vi "Hi_Tec_Control.vi"(0 "Carrier 1 Voltage":dbl(knob) min=0.0 max=5.0 scale=0.0..5.0 scale format="%.1f", 1 "Carrier 2 Voltage":dbl(knob) min=0.0 max=5.0 scale=0.0..5.0 scale format="%.1f", 2 "Trace Voltage":dbl(knob) min=0.0 max=5.0 scale=0.0..5.0 scale format="%.1f", 4 "Client Name":string) -> (5 "Scan Comments":string)   [LabVIEW 2014]
uses:
  Anemometry/Anemometry Sub Vis/Controls/In_Range.ctl
  ADAM Client/Sub VIs/ADAM Controls/Update_scan_value.ctl
panel:
  out "Second stage":dbl[][](graph)
  out "First stage":dbl[][](graph)
  out "Increasing trace":bool
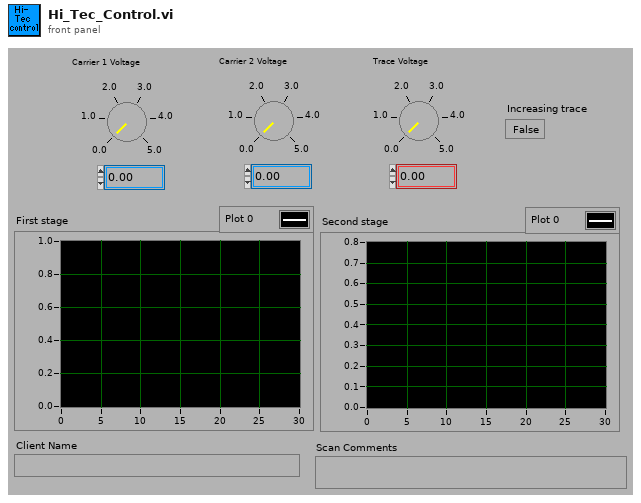
[diagram p1: front panel]
types:
  T1 = typedef "In_Range.ctl" = enum16{"%", "±", "% & ±"}
  T2 = typedef "Update_scan_value.ctl" = cluster{"Channel Name":string, "New Value":dbl}
  T3 = enum16{"Append to Global", "Read Global then Clear"}
  T4 = typedef "Ch_description_ADAM.ctl" = cluster{"Ch Name":string, "Type":T5, "Function":T6, "Ch State":T7, "Calibration type":T8, "A":dbl, "B":dbl, "C":dbl, "D":dbl, "Comments":string, "Address":T9, "String":string, "Duty":u16}
  T5 = typedef "Module_type_ADAM.ctl" = string
  T6 = typedef "Function_ADAM.ctl" = enum16{"Analogue Input", "Digital Input", "Event counter", "Event rate", "Analogue Output", "Digital Output", "Relay Output"}
  T7 = typedef "Channel_State.ctl" = enum16{"On", "Off", "Always On", "Always Off"}
  T8 = typedef "Calib_type_ADAM.ctl" = enum16{"Raw", "Bx + A", "Cx^2 + Bx + A", "Dx^3 + Cx^2 + Bx + A", "In Band", "Hi-Tec Q", "Hi-Tec M_dot", "Text"}
  T9 = typedef "Address.ctl" = cluster{"Main":i32, "Ch.":i32, "Sub":i32, "Port Name":string}
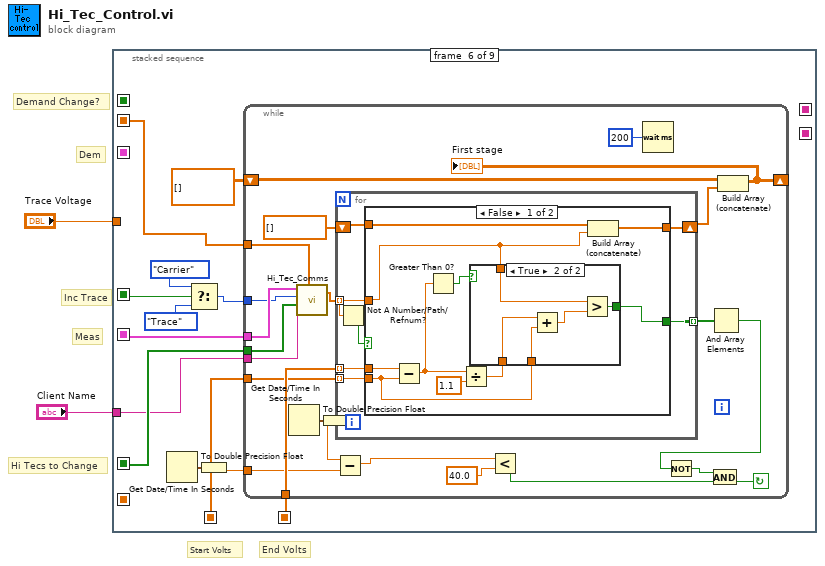
[diagram p0: block diagram]
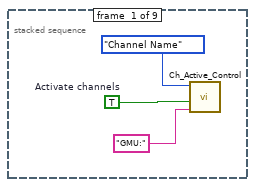
[diagram p2: hidden frame]
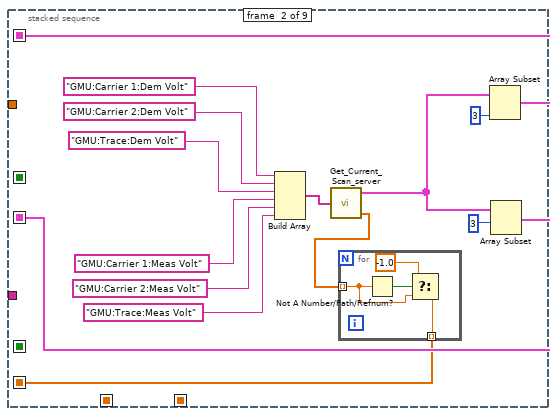
[diagram p3: hidden frame]
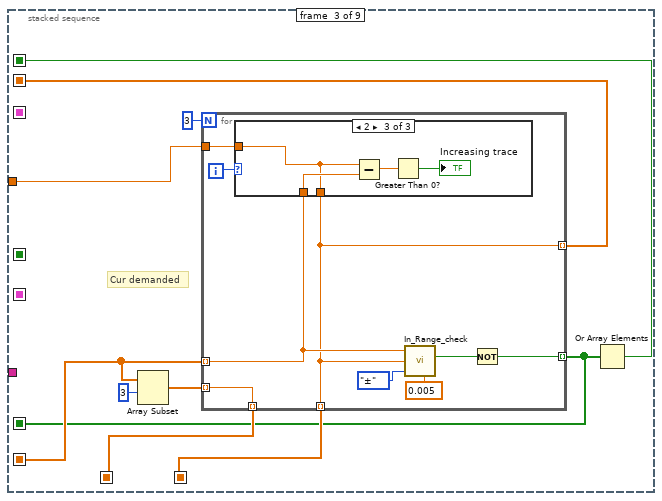
[diagram p4: hidden frame]
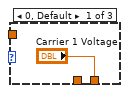
[diagram p5: hidden frame]
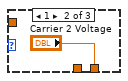
[diagram p6: hidden frame]
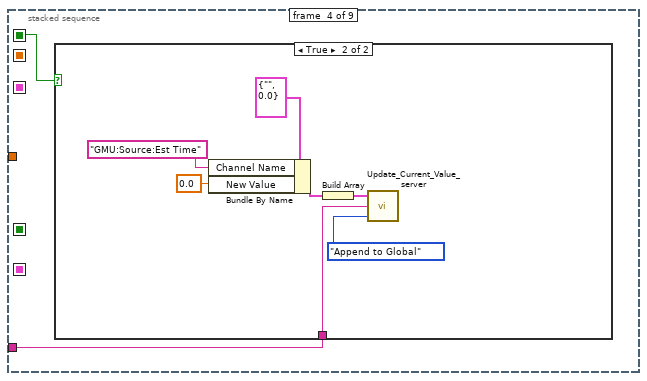
[diagram p7: hidden frame]
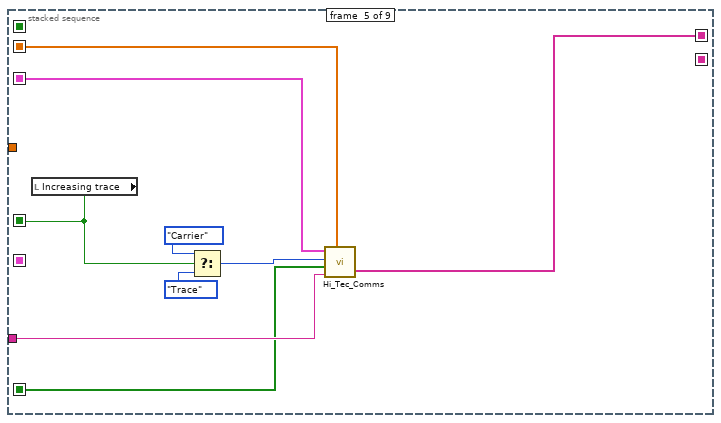
[diagram p9: hidden frame]
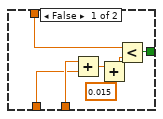
[diagram p10: hidden frame]
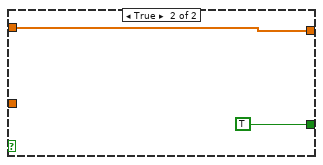
[diagram p11: hidden frame]
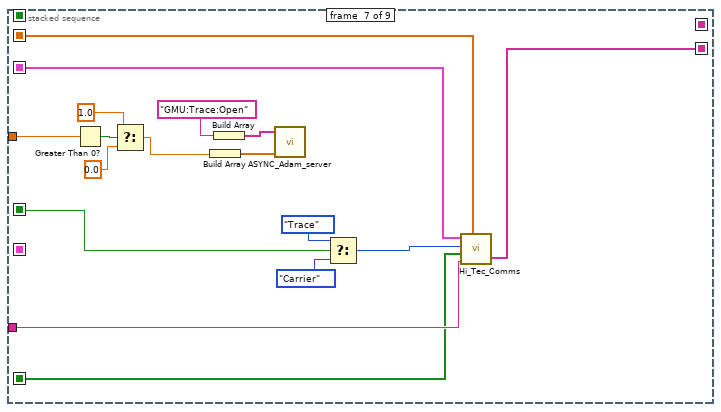
[diagram p12: hidden frame]
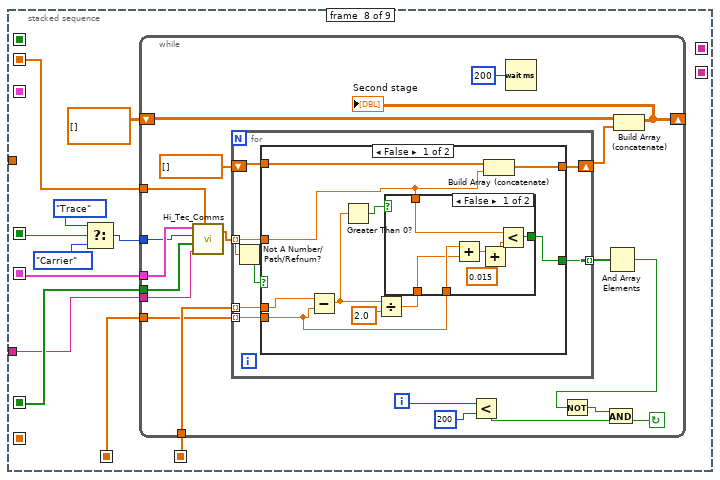
[diagram p13: hidden frame]
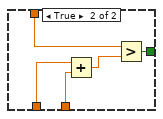
[diagram p14: hidden frame]
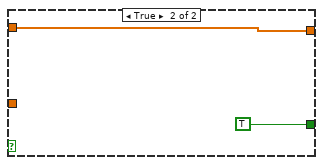
[diagram p15: hidden frame]
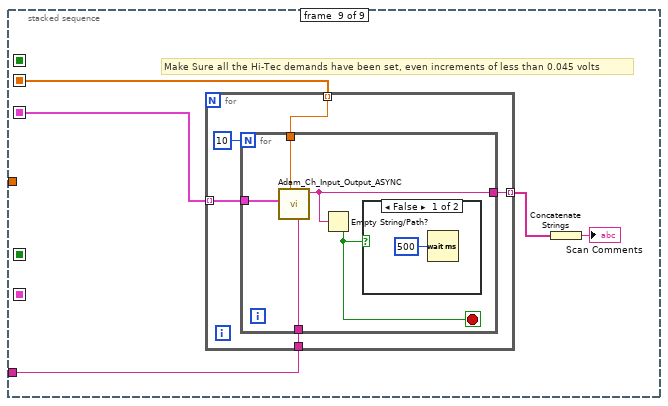
[diagram p16: hidden frame]
diagram:
  # "Dem"
  # "Demand Change?"
  # "End Volts"
  # "Start Volts"
  # "Inc Trace"
  # "Meas"
  # "Hi Tecs to Change"
  n1 = stacked-sequence {
    seq-local: [_ w14 _ _ _ _ _ _ _] -> [_ _ _ _ w60 _ w136 _ w216]
    seq-local: [_ w6 _ _ _ _ _ _ _] -> [_ _ w30 _ _ _ _ _ _]
    seq-local: [_ _ w27 _ _ _ _ _ _] -> [_ _ _ _ w59 w79 w135 w161 _]
    seq-local: [_ w13 _ _ _ _ _ _ _] -> [_ _ _ _ _ w75 _ w157 _]
    seq-local: [_ _ _ _ w66 _ _ _ _] -> [_ _ _ _ _ w76 w150 w158 _]
    seq-local: [_ _ w33 _ _ _ _ _ _] -> [_ _ _ _ _ w72 _ w154 _]
    seq-local: [_ _ w32 _ _ _ _ _ _] -> [_ _ _ _ _ w73 _ w155 _]
    seq-local: [_ _ w26 _ _ _ _ _ _] -> [_ _ _ w49 _ _ _ _ _]
    seq-local: [_ _ w24 _ _ _ _ _ _] -> [_ _ _ _ w61 w67 w137 w151 w215]
    seq-local: [_ _ _ _ w58 _ _ _ _] -> [_ _ _ _ _ _ _ _ _]
    seq-local: [_ _ _ _ _ _ w134 _ _] -> [_ _ _ _ _ _ _ _ _]
    tunnel: "Client Name" -> [_ _ _ w50 w62 w69 w146 w152 w217]
    tunnel: "Trace Voltage" -> [_ _ w25 _ _ _ w145 _ _]
    frame #0 {
      w3 = TRUE  # Activate channels
      n2 = call "Ch_Active_Control.vi"("Match"="GMU:", "Activate Channels?"=w3, "Control on"=enum16{"Channel Name", "Main Address"}."Channel Name") -> ()  [unwired: 1 in, 2 out]
    }
    frame #1 {
      n3 = Build Array("GMU:Carrier 1:Dem Volt", "GMU:Carrier 2:Dem Volt", "GMU:Trace:Dem Volt", "GMU:Carrier 1:Meas Volt", "GMU:Carrier 2:Meas Volt", "GMU:Trace:Meas Volt") -> (w19:string[])
      n4 = call "Get_Current_Scan_server.vi"("Desired Channels"=w19) -> ("Ch Description Array"=w12:T4[], "Numerical Values"=w7:dbl[])  [unwired: 1 out]
      n5 = for {
        tunnel: w7 -> [w22] mode=indexing
        tunnel: [w21] -> w6 mode=indexing
        n6 = Not A Number/Path/Refnum?(number/path/refnum=w22) -> (NaN/Path/Refnum?=w23:bool)
        n7 = Select(t=-1.0, s=w23, f=w22) -> (s? t:f=w21:dbl)
      }
      n8 = Array Subset(array=w12, length=3 ("Array Length")) -> (w14:T4[])  [unwired: 1 in]
      n9 = Array Subset(array=w12, index=3 ("Array Length")) -> (w13:T4[])  [unwired: 1 in]
    }
    frame #2 {
      # "Cur demanded"
      n10 = Array Subset(array=w30, index=3 ("Array Index")) -> (w28:dbl[])  [unwired: 1 in]
      n11 = for {
        N: 3 -> [_]
        tunnel: w30 -> [w37] mode=indexing
        tunnel: [w40] -> w33 mode=indexing
        tunnel: [w34] -> w32 mode=indexing
        tunnel: [w41] -> w27 mode=indexing
        tunnel: w28 -> [w40] mode=indexing
        tunnel: w25 -> [w35]
        tunnel: [w34] -> w24 mode=indexing
        i -> [w42]
        n12 = case shown="2" w42 {
          tunnel: ["Carrier 1 Voltage" "Carrier 2 Voltage" w45] -> w34
          tunnel: w37 -> [_ _ w48]
          tunnel: w35 -> [_ _ w45]
          frame 0, Default {
          }
          frame 1 {
          }
          frame 2 {
            n13 = Subtract(x=w45, y=w48) -> (x-y=w47:dbl)
            n14 = Greater Than 0?(x=w47) -> (x > 0?=→"Increasing trace":bool)
          }
        }
        n15 = call "In_Range_check.vi"("±"=0.005 ("%"), "Mode"=In_Range."±", "Value"=w34, "Setpoint"=w37) -> ("In Range"=w36:bool)  [unwired: 1 in, 2 out]
        n16 = Not(x=w36) -> (.not. x?=w41:bool)
      }
      n17 = Or Array Elements(Boolean array=w27) -> (logical OR=w26:bool)
    }
    frame #3 {
      n18 = case shown="True" w49 {
        tunnel: w50 -> [_ w57]
        frame False {
        }
        frame True {
          n19 = Bundle By Name(cluster=T2 {"Channel Name"="", "New Value"=0.0} ("Update Scan Value Cluster"), "Channel Name"="GMU:Source:Est Time", "New Value"=0.0 ("Bundle Element")) -> (w52:T2)
          n20 = Build Array(w52) -> (w51:T2[])
          n21 = call "Update_Current_Value_server.vi"("Mode"=T3."Append to Global", "Client HD name"=w57, "Update array in"=w51) -> ()  [unwired: 1 out]
        }
      }
    }
    frame #4 {
      n22 = local read "Increasing trace"() -> (w66:bool)
      n23 = Select(t=enum16{"Carrier", "Trace"}."Carrier" ("Type"), s=w66, f=enum16{"Carrier", "Trace"}."Trace" ("Type")) -> (s? t:f=w63:enum16{"Carrier", "Trace"})
      n24 = call "Hi_Tec_Comms.vi"("Ch Description Array"=w60, "Type"=w63, "Hi Tec's To Change"=w59, "Client Name"=w62, "Dem Volts"=w61) -> ("Scan comments"=w58:string[])  [unwired: 1 out]
    }
    frame #5 {
      n25 = Get Date/Time In Seconds() -> (seconds since 1Jan1904=w68:timestamp)
      n26 = Select(t=enum16{"Carrier", "Trace"}."Carrier" ("Type"), s=w76, f=enum16{"Carrier", "Trace"}."Trace" ("Type")) -> (s? t:f=w74:enum16{"Carrier", "Trace"})
      n27 = To Double Precision Float(number=w68) -> (double precision float=w70:dbl)
      n28 = while {
        tunnel: w69 -> [w83]
        tunnel: w70 -> [w86]
        shift-left: dbl[][] [] -> [w92]
        shift-right: [w91] -> _
        tunnel: w72 -> [w99]
        tunnel: w73 -> [w100]
        tunnel: w74 -> [w101]
        tunnel: w75 -> [w102]
        tunnel: w79 -> [w93]
        tunnel: w67 -> [w80]
        stop <- w88 continue-if-true
        n29 = Get Date/Time In Seconds() -> (seconds since 1Jan1904=w82:timestamp)
        n30 = call "Hi_Tec_Comms.vi"("Ch Description Array"=w102, "Type"=w101, "Hi Tec's To Change"=w93, "Client Name"=w83, "Dem Volts"=w80) -> ("Outputs"=w98:dbl[])  [unwired: 1 out]
        n31 = To Double Precision Float(number=w82) -> (double precision float=w87:dbl)
        n32 = Subtract(x=w87, y=w86) -> (x-y=w85:dbl)
        n33 = for {
          tunnel: w100 -> [w109] mode=indexing
          tunnel: w99 -> [w108] mode=indexing
          tunnel: w98 -> [w104] mode=indexing
          tunnel: [w107] -> w97 mode=indexing
          shift-right: [w105] -> w94
          shift-left: dbl[] [] -> [w106]
          n34 = Not A Number/Path/Refnum?(number/path/refnum=w104) -> (NaN/Path/Refnum?=w103:bool)
          n35 = case shown="False" w103 {
            tunnel: w109 -> [w116 _]
            tunnel: w108 -> [w112 _]
            tunnel: w104 -> [w111 _]
            tunnel: [w110 TRUE] -> w107
            tunnel: w106 -> [w115 w132]
            tunnel: [w114 w132] -> w105
            frame False {
              n36 = Subtract(x=w116, y=w112) -> (x-y=w118:dbl)
              n37 = Greater Than 0?(x=w118) -> (x > 0?=w117:bool)
              n38 = Divide(x=w118, y=1.1) -> (x/y=w113:dbl)
              n39 = case shown="True" w117 {
                tunnel: w113 -> [w125 w131]
                tunnel: w112 -> [w126 w130]
                tunnel: w111 -> [w124 w128]
                tunnel: [w123 w127] -> w110
                frame False {
                  n40 = Add(x=w126, y=w125) -> (x+y=w122:dbl)
                  n41 = Add(x=w122, y=0.015 ("x")) -> (x+y=w121:dbl)
                  n42 = Less?(x=w124, y=w121) -> (x < y?=w123:bool)
                }
                frame True {
                  n43 = Add(x=w131, y=w130) -> (x+y=w129:dbl)
                  n44 = Greater?(x=w128, y=w129) -> (0:w127:bool)
                }
              }
              n45 = Build Array (concatenate)(w115, w111) -> (w114:dbl[])
            }
            frame True {
            }
          }
        }
        n46 = Less?(x=w85, y=40.0) -> (x < y?=w90:bool)
        n47 = Wait (ms)(milliseconds to wait=u32 200) -> ()  [unwired: 1 out]
        n48 = And Array Elements(Boolean array=w97) -> (logical AND=w96:bool)
        n49 = Not(x=w96) -> (.not. x?=w89:bool)
        n50 = And(x=w89, y=w90) -> (x .and. y?=w88:bool)
        n51 = Build Array (concatenate)(w92, w94) -> (w91:dbl[][])
        "First stage" <- w91
      }
    }
    frame #6 {
      n52 = Greater Than 0?(x=w145) -> (x > 0?=w144:bool)
      n53 = Select(t=1.0, s=w144, f=0.0) -> (s? t:f=w141:dbl)
      n54 = Build Array(w141) -> (w138:dbl[])
      n55 = Build Array("GMU:Trace:Open") -> (w139:string[])
      n56 = call "ASYNC_Adam_server.vi"("Values"=w138, "Channel Names"=w139) -> ()  [unwired: 2 in, 2 out]
      n57 = Select(t=enum16{"Carrier", "Trace"}."Trace" ("Type"), s=w150, f=enum16{"Carrier", "Trace"}."Carrier" ("Type")) -> (s? t:f=w147:enum16{"Carrier", "Trace"})
      n58 = call "Hi_Tec_Comms.vi"("Ch Description Array"=w136, "Type"=w147, "Hi Tec's To Change"=w135, "Client Name"=w146, "Dem Volts"=w137) -> ("Scan comments"=w134:string[])  [unwired: 1 out]
    }
    frame #7 {
      n59 = Select(t=enum16{"Carrier", "Trace"}."Trace" ("Type"), s=w158, f=enum16{"Carrier", "Trace"}."Carrier" ("Type")) -> (s? t:f=w156:enum16{"Carrier", "Trace"})
      n60 = while {
        tunnel: w152 -> [w164]
        shift-left: dbl[][] [] -> [w171]
        shift-right: [w165] -> _
        tunnel: w154 -> [w178]
        tunnel: w155 -> [w179]
        tunnel: w156 -> [w180]
        tunnel: w157 -> [w181]
        tunnel: w161 -> [w172]
        tunnel: w151 -> [w162]
        i -> [w167]
        stop <- w166 continue-if-true
        n61 = call "Hi_Tec_Comms.vi"("Ch Description Array"=w181, "Type"=w180, "Hi Tec's To Change"=w172, "Client Name"=w164, "Dem Volts"=w162) -> ("Outputs"=w177:dbl[])  [unwired: 1 out]
        n62 = for {
          tunnel: w179 -> [w188] mode=indexing
          tunnel: w178 -> [w187] mode=indexing
          tunnel: w177 -> [w183] mode=indexing
          tunnel: [w186] -> w176 mode=indexing
          shift-right: [w184] -> w173
          shift-left: dbl[] [] -> [w185]
          n63 = Not A Number/Path/Refnum?(number/path/refnum=w183) -> (NaN/Path/Refnum?=w182:bool)
          n64 = case shown="False" w182 {
            tunnel: w188 -> [w192 _]
            tunnel: w187 -> [w191 _]
            tunnel: w183 -> [w190 _]
            tunnel: [w189 TRUE] -> w186
            tunnel: w185 -> [w198 w211]
            tunnel: [w197 w211] -> w184
            frame False {
              n65 = Subtract(x=w192, y=w191) -> (x-y=w195:dbl)
              n66 = Greater Than 0?(x=w195) -> (x > 0?=w194:bool)
              n67 = Divide(x=w195, y=2.0) -> (x/y=w193:dbl)
              n68 = case shown="False" w194 {
                tunnel: w193 -> [w204 w210]
                tunnel: w191 -> [w205 w209]
                tunnel: w190 -> [w203 w207]
                tunnel: [w202 w206] -> w189
                frame False {
                  n69 = Add(x=w205, y=w204) -> (x+y=w201:dbl)
                  n70 = Add(x=w201, y=0.015 ("x")) -> (x+y=w200:dbl)
                  n71 = Less?(x=w203, y=w200) -> (x < y?=w202:bool)
                }
                frame True {
                  n72 = Add(x=w210, y=w209) -> (x+y=w208:dbl)
                  n73 = Greater?(x=w207, y=w208) -> (0:w206:bool)
                }
              }
              n74 = Build Array (concatenate)(w198, w190) -> (w197:dbl[])
            }
            frame True {
            }
          }
        }
        n75 = Less?(x=w167, y=200) -> (x < y?=w169:bool)
        n76 = Wait (ms)(milliseconds to wait=u32 200) -> ()  [unwired: 1 out]
        n77 = And Array Elements(Boolean array=w176) -> (logical AND=w175:bool)
        n78 = Not(x=w175) -> (.not. x?=w168:bool)
        n79 = And(x=w168, y=w169) -> (x .and. y?=w166:bool)
        n80 = Build Array (concatenate)(w171, w173) -> (w165:dbl[][])
        "Second stage" <- w165
      }
    }
    frame #8 {
      # "Make Sure all the Hi-Tec demands have been set, even increments of less than 0.045 volts"
      n81 = for {
        tunnel: w216 -> [w222] mode=indexing
        tunnel: w217 -> [w220]
        tunnel: w215 -> [w221] mode=indexing
        tunnel: [w219] -> w214 mode=indexing
        n82 = for {
          N: 10 -> [_]
          tunnel: w222 -> [w227]
          tunnel: w221 -> [w226]
          tunnel: w220 -> [w225]
          tunnel: [w224] -> w219
          stop <- w223 stop-if-true
          n83 = call "Adam_Ch_Input_Output_ASYNC.vi"("Client Name"=w225, "Value to Output"=w226, "Ch Discription"=w227) -> ("Scan comment"=w224:string)  [unwired: 4 in, 4 out]
          n84 = Empty String/Path?(string/path=w224) -> (empty?=w223:bool)
          n85 = case shown="False" w223 {
            frame False {
              n86 = Wait (ms)(milliseconds to wait=u32 500) -> ()  [unwired: 1 out]
            }
            frame True {
            }
          }
        }
      }
      n87 = Concatenate Strings(w214) -> (→"Scan Comments":string)
    }
  }
